vi "Match VIs Ctls.vi"(7 "Calling VI Ref":refnum<vi>, 8 "Error In":errorcluster, 9 "Traverse Clusters (F)":bool=TRUE, 10 "Ctls Refs (All Ctls)":refnum<vi>[](array[refnum]), 11 "VI Ref":refnum<vi>) -> (0 "Error Out":errorcluster, 2 "Matching Ctls Out":refnum<vi>[](array[refnum]), 3 "Used Panel":refnum<vi>)   [LabVIEW 2020, in "UIM.lvlib" / "UIM.lvclass"]
doc: "Output only the ctrl references that are in both arrays. If the wired input is empty, return all VIs ctls refs."
uses:
  UIM.lvclass
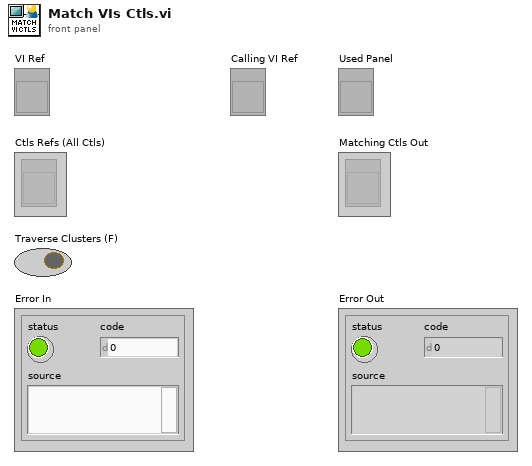
[diagram p1: front panel]
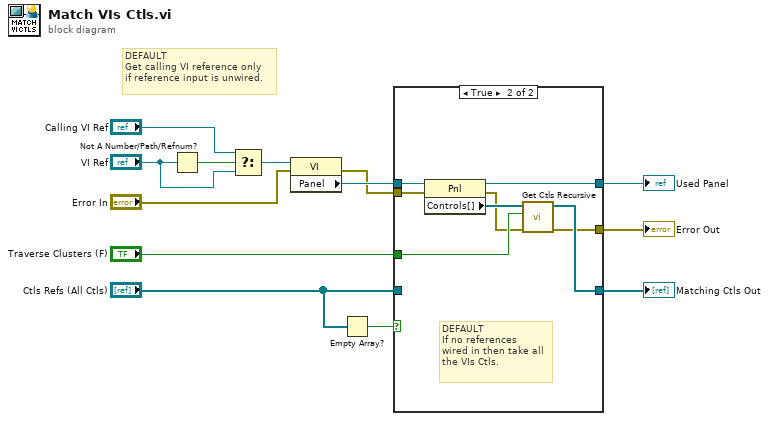
[diagram p0: block diagram]
diagram:
  # "DEFAULT\nGet calling VI reference only \nif reference input is unwired."
  n1 = Not A Number/Path/Refnum?(number/path/refnum="VI Ref") -> (NaN/Path/Refnum?=w10:bool)
  n2 = Select(t="Calling VI Ref", s=w10, f="VI Ref") -> (s? t:f=w11:refnum<vi>)
  n3 = property class="VI"(reference=w11, error in="Error In") -> (error out=w1:errorcluster, "Panel"=w5:refnum<vi>)  [unwired: 1 out]
  n4 = Empty Array?(array="Ctls Refs (All Ctls)") -> (empty?=w8:bool)
  n5 = case shown="True" w8 {
    tunnel: "Ctls Refs (All Ctls)" -> [w16 _]
    tunnel: [w16 w21] -> w6
    tunnel: w5 -> [w15 w23]
    tunnel: [w15 w22] -> w4
    tunnel: "Traverse Clusters (F)" -> [_ w20]
    tunnel: [w14 w18] -> w2
    tunnel: w1 -> [w14 w17]
    frame False {
    }
    frame True {
      # "DEFAULT\nIf no references \nwired in then take all\nthe VIs Ctls."
      n6 = property class="Pnl"(reference=w23, error in=w17) -> (reference out=w22:refnum<vi>, error out=w19:errorcluster, "Controls[]"=w24:refnum<vi>[])
      n7 = call "Get Ctls Recursive.vi"("Error In"=w19, "Traverse Clusters (F)"=w20, "Ctls"=w24) -> ("Error Out"=w18:errorcluster, "Recursive All Ctls"=w21:refnum<vi>[])  [unwired: 7 in]
    }
  }
  "Error Out" <- w2
  "Matching Ctls Out" <- w6
  "Used Panel" <- w4
